vi "NF LI56xx dvr MEMory STATe DEFine.vi"(8 "error in":errorcluster caption="error in (no error)" {"code" format="%.0x"}, 9 "Read(F)":bool, 10 "set memory No.":u8=1 min=1 max=9 step=1, 11 "VISA resource name":refnum<visa-resource-name>) -> (0 "error out":errorcluster {"code" format="%.0x"}, 2 "query memory name":string, 3 "VISA resource name copy":refnum<visa-resource-name>)   [LabVIEW 2019]
doc: "Changes the name of the specified configuration memory. \nAlso queries the memory name of the specified configuration memory."
panel:
  in  "set memory name":string
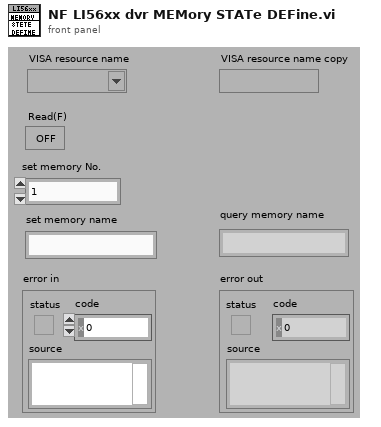
[diagram p1: front panel]
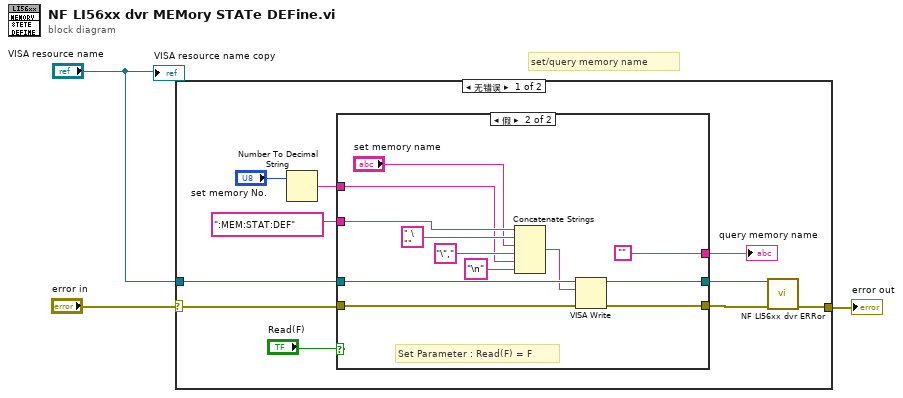
[diagram p0: block diagram]
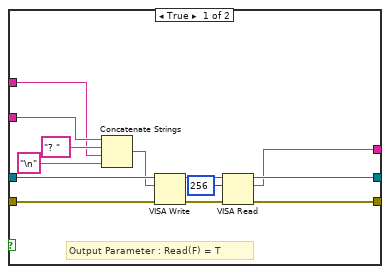
[diagram p2: hidden frame]
diagram:
  # "set/query memory name"
  n1 = case shown="无错误" "error in" {
    selector: "error in" -> [w12 w39]
    tunnel: [w7 w39] -> w3
    tunnel: "VISA resource name" -> [w11 _]
    frame No Error {
      n2 = Number To Decimal String(number="set memory No.") -> (decimal integer string=w4:string)  [unwired: 1 in]
      n3 = case shown="假" "Read(F)" {
        tunnel: w11 -> [w26 w38]
        tunnel: [w23 w35] -> w9
        tunnel: [w22 w36] -> w8
        tunnel: w12 -> [w21 w37]
        tunnel: [w17 ""] -> w10
        tunnel: ":MEM:STAT:DEF" ("•¶Žš—ñ") -> [w16 w32]
        tunnel: w4 -> [w15 w28]
        frame True {
          # "Output Parameter : Read(F) = T"
          n4 = Concatenate Strings(w16, "? " ("Œ`Ž®•¶Žš—ñ"), w15, "\n" ("Œ`Ž®•¶Žš—ñ")) -> (w18:string)
          n5 = VISA Write(VISA resource name=w26, write buffer=w18, error in (no error)=w21) -> (VISA resource name out=w24:refnum<visa-resource-name>, error out=w25:errorcluster)  [unwired: 1 out]
          n6 = VISA Read(VISA resource name=w24, byte count=u32 256 ("バイトカウント（0）"), error in (no error)=w25) -> (VISA resource name out=w23:refnum<visa-resource-name>, read buffer=w17:string, error out=w22:errorcluster)  [unwired: 1 out]
        }
        frame False {
          # "Set Parameter : Read(F) = F"
          n7 = Concatenate Strings(w32, " \"", "set memory name", "\",", w28, "\n" ("Œ`Ž®•¶Žš—ñ")) -> (w33:string)
          n8 = VISA Write(VISA resource name=w38, write buffer=w33, error in (no error)=w37) -> (VISA resource name out=w35:refnum<visa-resource-name>, error out=w36:errorcluster)  [unwired: 1 out]
        }
      }
      "query memory name" <- w10
      n9 = call "NF LI56xx dvr ERRor.vi"("VISA resource name"=w9, "error in (no error)"=w8) -> ("error out"=w7:errorcluster)  [unwired: 10 in, 3 out]
    }
    frame Error {
    }
  }
  "error out" <- w3
  "VISA resource name copy" <- "VISA resource name"
